vi "Project Dir.vi"(8 "error in (no error)":errorcluster) -> (0 "error out":errorcluster, 3 "path":path)   [LabVIEW 2014, in "lvprj2html.lvlib"]
uses:
  lvprj2html.lvlib
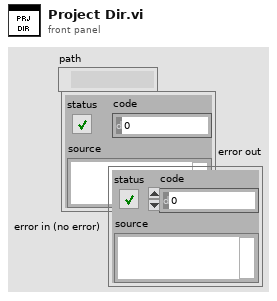
[diagram p1: front panel]
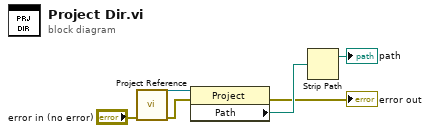
[diagram p0: block diagram]
diagram:
  n1 = call "Project Reference.vi"("error in (no error)"="error in (no error)") -> ("error out"=w3:errorcluster, "prj ref"=w5:refnum<vi>)  [unwired: 9 in]
  n2 = property class="Project"(reference=w5, error in=w3) -> (error out=→"error out":errorcluster, "Path"=w4:path)  [unwired: 1 out]
  n3 = Strip Path(path=w4) -> (stripped path=→"path":path)  [unwired: 1 out]
